vi "subXMLGetSourceItemInclusion.vi"(9 "index (1)":u32=1, 11 "Refnum in":refnum<k20>) -> (3 "Include?":bool)   [LabVIEW 2019, in "SolutionBuilder.lvlib" / "SolutionBuilder.lvclass"]
uses:
  SolutionBuilder.lvclass
  <vilib>/xml/NI_XML.lvlib
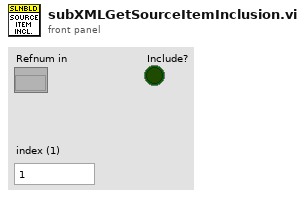
[diagram p1: front panel]
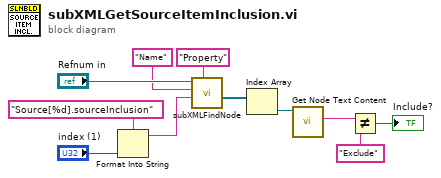
[diagram p0: block diagram]
diagram:
  n1 = Format Into String(format string="Source[%d].sourceInclusion" ("Property value"), "index (1)") -> (resulting string=w5:string)  [unwired: 2 in, 1 out]
  n2 = call "subXMLFindNode.vi"("Node name"="Property", "Property value"=w5, "Property name"="Name", "Refnum in"="Refnum in") -> ("Nodes"=w9:refnum<k20>[])  [unwired: 6 in, 1 out]
  n3 = Index Array(array=w9) -> (element=w10:refnum<k20>)  [unwired: 1 in]
  n4 = call <vilib>:"Get Node Text Content.vi"("node in"=w10) -> ("node text"=w3:string)  [unwired: 8 in, 2 out]
  n5 = Not Equal?(x=w3, y="Exclude" ("regular expression")) -> (x != y?=→"Include?":bool)
